vi "NI 5772 (AC) - Digitizer_(FPGA)Averaging (Working)BeforeEdits.vi"() -> ()   [LabVIEW 2020]
doc: "Example Description:\nThis example demonstrates how to enable Time Interleaved Sampling with the NI 5772 adapter module to achieve a sampling rate of 1.6GS/s. This example continuously acquires records of analog input data from the NI 5772 adapter module. It allows you to select an AI channel, trigger type, and record size. This VI must be compiled before it is run. \n\nRunning the VI:\nThis VI must be run from the NI 5772 - Getting Started (Host).vi. Refer to the host VI documentation for steps regarding running and configuring the FPGA VI. \n\nExecution Steps:\nRefer to the Block Diagram of this VI for execution comments."
uses:
  Controls/AI Trigger Type.ctl
  Controls/Aquire State.ctl
  <vilib>/Platform/TimedLoop/XDataNode/timing_clust.ctl
  <vilib>/Platform/TimedLoop/XDataNode/nitl_modes.ctl
  <vilib>/Platform/TimedLoop/XDataNode/wakeup.ctl
  Controls/DigitizerState.ctl
  <vilib>/rvi/Emulation/niFpgaGetClockAttributes.vi
  <vilib>/rvi/Emulation/niFpgaSctlEmulationGetInTimedLoop.vi
  <vilib>/rvi/Emulation/niFpgaEmulationReportErrorSimple.vi
  <vilib>/rvi/eio/common/nirviEmuTemplateMethod_errors.vi
  <vilib>/rvi/Emulation/niFpgaCriticalErrorInLSC.vi
  <vilib>/rvi/Emulation/niFpgaProcessEmulError.vi
  <vilib>/rvi/Emulation/niFpgaEmulationIsFPGAContextNoSignature.vi
  <vilib>/rvi/errors/niFpgaSetErrorForExecOnDevCompSimple.vi
  <vilib>/rvi/eio/common/nirviEmuReportErrorAndStop.vi
  <vilib>/rvi/DataTransferAndStorage/Container/Common/niFpgaContainerGetUniqueNameForEmu.vi
  <vilib>/rvi/FIFO/Fifo_Resource/nirvififoEmulationSetSize.vi
  <vilib>/rvi/FIFO/Fifo_Resource/nirviFifoEmulationQueueMgr.vi
  <instcachedir>/0/nirviFifoEmulationQueueMgr_E5CAEC123FF24DC58D834DCA3CDAA9B5.lvgen/nirviFifoEmulationQueueMgr_E5CAEC123FF24DC58D834DCA3CDAA9B5_000.vi
  <vilib>/Utility/error.llb/Clear Errors.vi
  <vilib>/rvi/FIFO/Fifo_Resource/nirvififoEmulationCreateLock.vi
  <vilib>/rvi/FIFO/Fifo_Resource/nirvififoEmulationObtainLock.vi
  <vilib>/rvi/FIFO/Fifo_Resource/nirvififoEmulationReleaseLock.vi
  <vilib>/rvi/occurrence/nirviWaitOnOccurrenceBase.vi
  <vilib>/rvi/errors/nirviReportUnexpectedCaseInternalError.vi
  <vilib>/rvi/errors/nirviReportUnexpectedCaseInternalError (U32).vi
  <instcachedir>/0/nirviFifoEmulationQueueMgr_E5CAEC123FF24DC58D834DCA3CDAA9B5.lvgen/nirviFifoEmulationQueueMgr_E5CAEC123FF24DC58D834DCA3CDAA9B5_003.vi
  <vilib>/rvi/FIFO/Fifo_Resource/nirvififoEmulationDetermineInputValidOut.vi
  <vilib>/rvi/Memory/Memory_Emulation/nirvimemoryFastEmulation.vi
  <vilib>/rvi/Memory/Memory_Emulation/nirvimemoryEmulation.vi
  <vilib>/rvi/interface/RandomDataEmulation/niFpgaRandomDataHandleErrors.vi
  <instcachedir>/0/nirviFifoEmulationQueueMgr_E5CAEC123FF24DC58D834DCA3CDAA9B5.lvgen/nirviFifoEmulationQueueMgr_E5CAEC123FF24DC58D834DCA3CDAA9B5_004.vi
  <vilib>/eio/EIONode/EIONode.xnode
  <vilib>/Platform/TimedLoop/XDataNode/XDataNode.xnode
  <vilib>/rvi/DataTransferAndStorage/Container/XNode/niFpgaContainer.xnode
  <vilib>/rvi/FIFO/Fifo_Resource/nirvififoEmulationRead.vi
  <vilib>/rvi/FIFO/Fifo_Resource/nirvififoEmulationWrite.vi
  <vilib>/rvi/interface/RandomDataEmulation/nirviRandomDataFpgaReadWriteTemplate.vi
  <vilib>/Platform/TimedLoop/XDataNode/XDNodeRunTimeDep.lvlib
  <instrlib>/_niInstr/Basic Elements/v1/FPGA/niInstr Basic Elements v1 FPGA.lvlib
  <instrlib>/_niInstr/Basic Elements/v1/FPGA/Private/Count Up U64.vi
panel:
  in  "Pulse Width [cycles]":u16=5
  out "Align Wave Counter":u64
  out "Read Size (Host)":u16=512 caption="Samples Per Trigger" min=1 step=1
  out "Trig Count":u64
  in  "TrigIn Simulate":bool
  in  "vi/nGenTrig":bool
  in  "Arm Trigger":bool
  out "F to H FIFO Overflow?":bool caption="FIFO Overflow?"
  out "DataAlignmentFIFO":bool
  out "Aq to Trans FIFO Overflow?":bool caption="FIFO Overflow?"
  in  "Requested Samples Per Pixel":u16=512 caption="Samples Per Trigger" min=1 step=1
  in  "AvgCount_powerOf2":i16=1
  in  "Delay (us)":sgl
  in  "WaveSampleCount":sgl=256.0 format="%#_13g"
  in  "Wave Sampling Rate":sgl=200000000.0 format="%#_6p"
  in  "Trigger Level":i16
  in  "Trigger Type":T1
  out "AvgCount":u16=1
  out "Delay after Trig [cycles]":u16
  out "1/8th Samples Per Trigger":u16=512 caption="Samples Per Trigger" min=1 step=1
  out "WaitForWave\nCompletion [cycles]":u16
  in  "User Command Commit":bool
  in  "User Command":u8
  out "User Command Idle":bool
  out "User Command Status":u8
  in  "User Data 0":u16
  in  "User Data 1":u8
  out "PLL Locked":bool
  out "User Error":bool
  out "Configured?":bool
  # "FIFO Status"
  # "Analog Input"
  # "Resource Configuration"
  # "Clock Configuration"
  # "Trigger Settings"
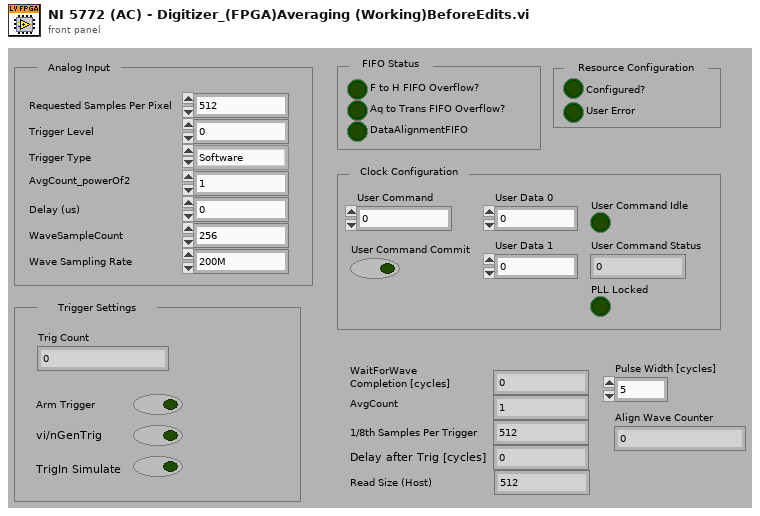
[diagram p1: front panel]
types:
  T1 = typedef "AI Trigger Type.ctl" = enum8{"Software", "Data Edge"}
  T2 = typedef "DigitizerState.ctl" = enum16{"Init", "Build/Clear Accumulator", "GetData", "SetData", "AverageCountCheck", "SendtoHost"}
  T3 = typedef "Aquire State.ctl" = enum8{"Idle", "Wait for Trigger", "AlignWave", "Hold Aquire", "Acquire", "WaitForWaveCompletion", "CheckAvg"}
  T4 = typedef "XDNodeRunTimeDep.lvlib/timing_clust.ctl" = cluster{"Expected End [f-1]":u64, "Actual End [f-1]":u64, "Finished Late? [f-1]":bool, "Expected End [i-1]":u64, "Actual End [i-1]":u64, "Finished Late? [i-1]":bool, "Expected Start [i]":u64, "Actual Start [i]":u64, "Expected Start [f]":u64, "Actual Start [f]":u64, "Source Name":string, "Structure Name":string, "Period":i64, "Deadline":i64, "Offset":i64, "Start":i64, "Priority":i32, "Timeout":i32, "Mode":T5, "Wakeup Reason":T6, "Error":errorcluster, "Source Type":string, "Secondary Source Type":string, "Global End Time":u64, "Global Start Time":u64, "Frame Duration":u64, "Iteration Duration":u64, "Assigned CPU":i32, "I/O Scan Engine Mode":u32}
  T5 = typedef "XDNodeRunTimeDep.lvlib/nitl_modes.ctl" = enum32{"No Change", "Process missed periods, maintain original phase", "Discard missed periods, maintain original phase", "Process missed periods, ignore original phase", "Discard missed periods, ignore original phase"}
  T6 = typedef "XDNodeRunTimeDep.lvlib/wakeup.ctl" = enum32{"Normal", "Aborted", "Asynchronous wakeup", "Timing source error", "Timed loop error", "Timeout"}
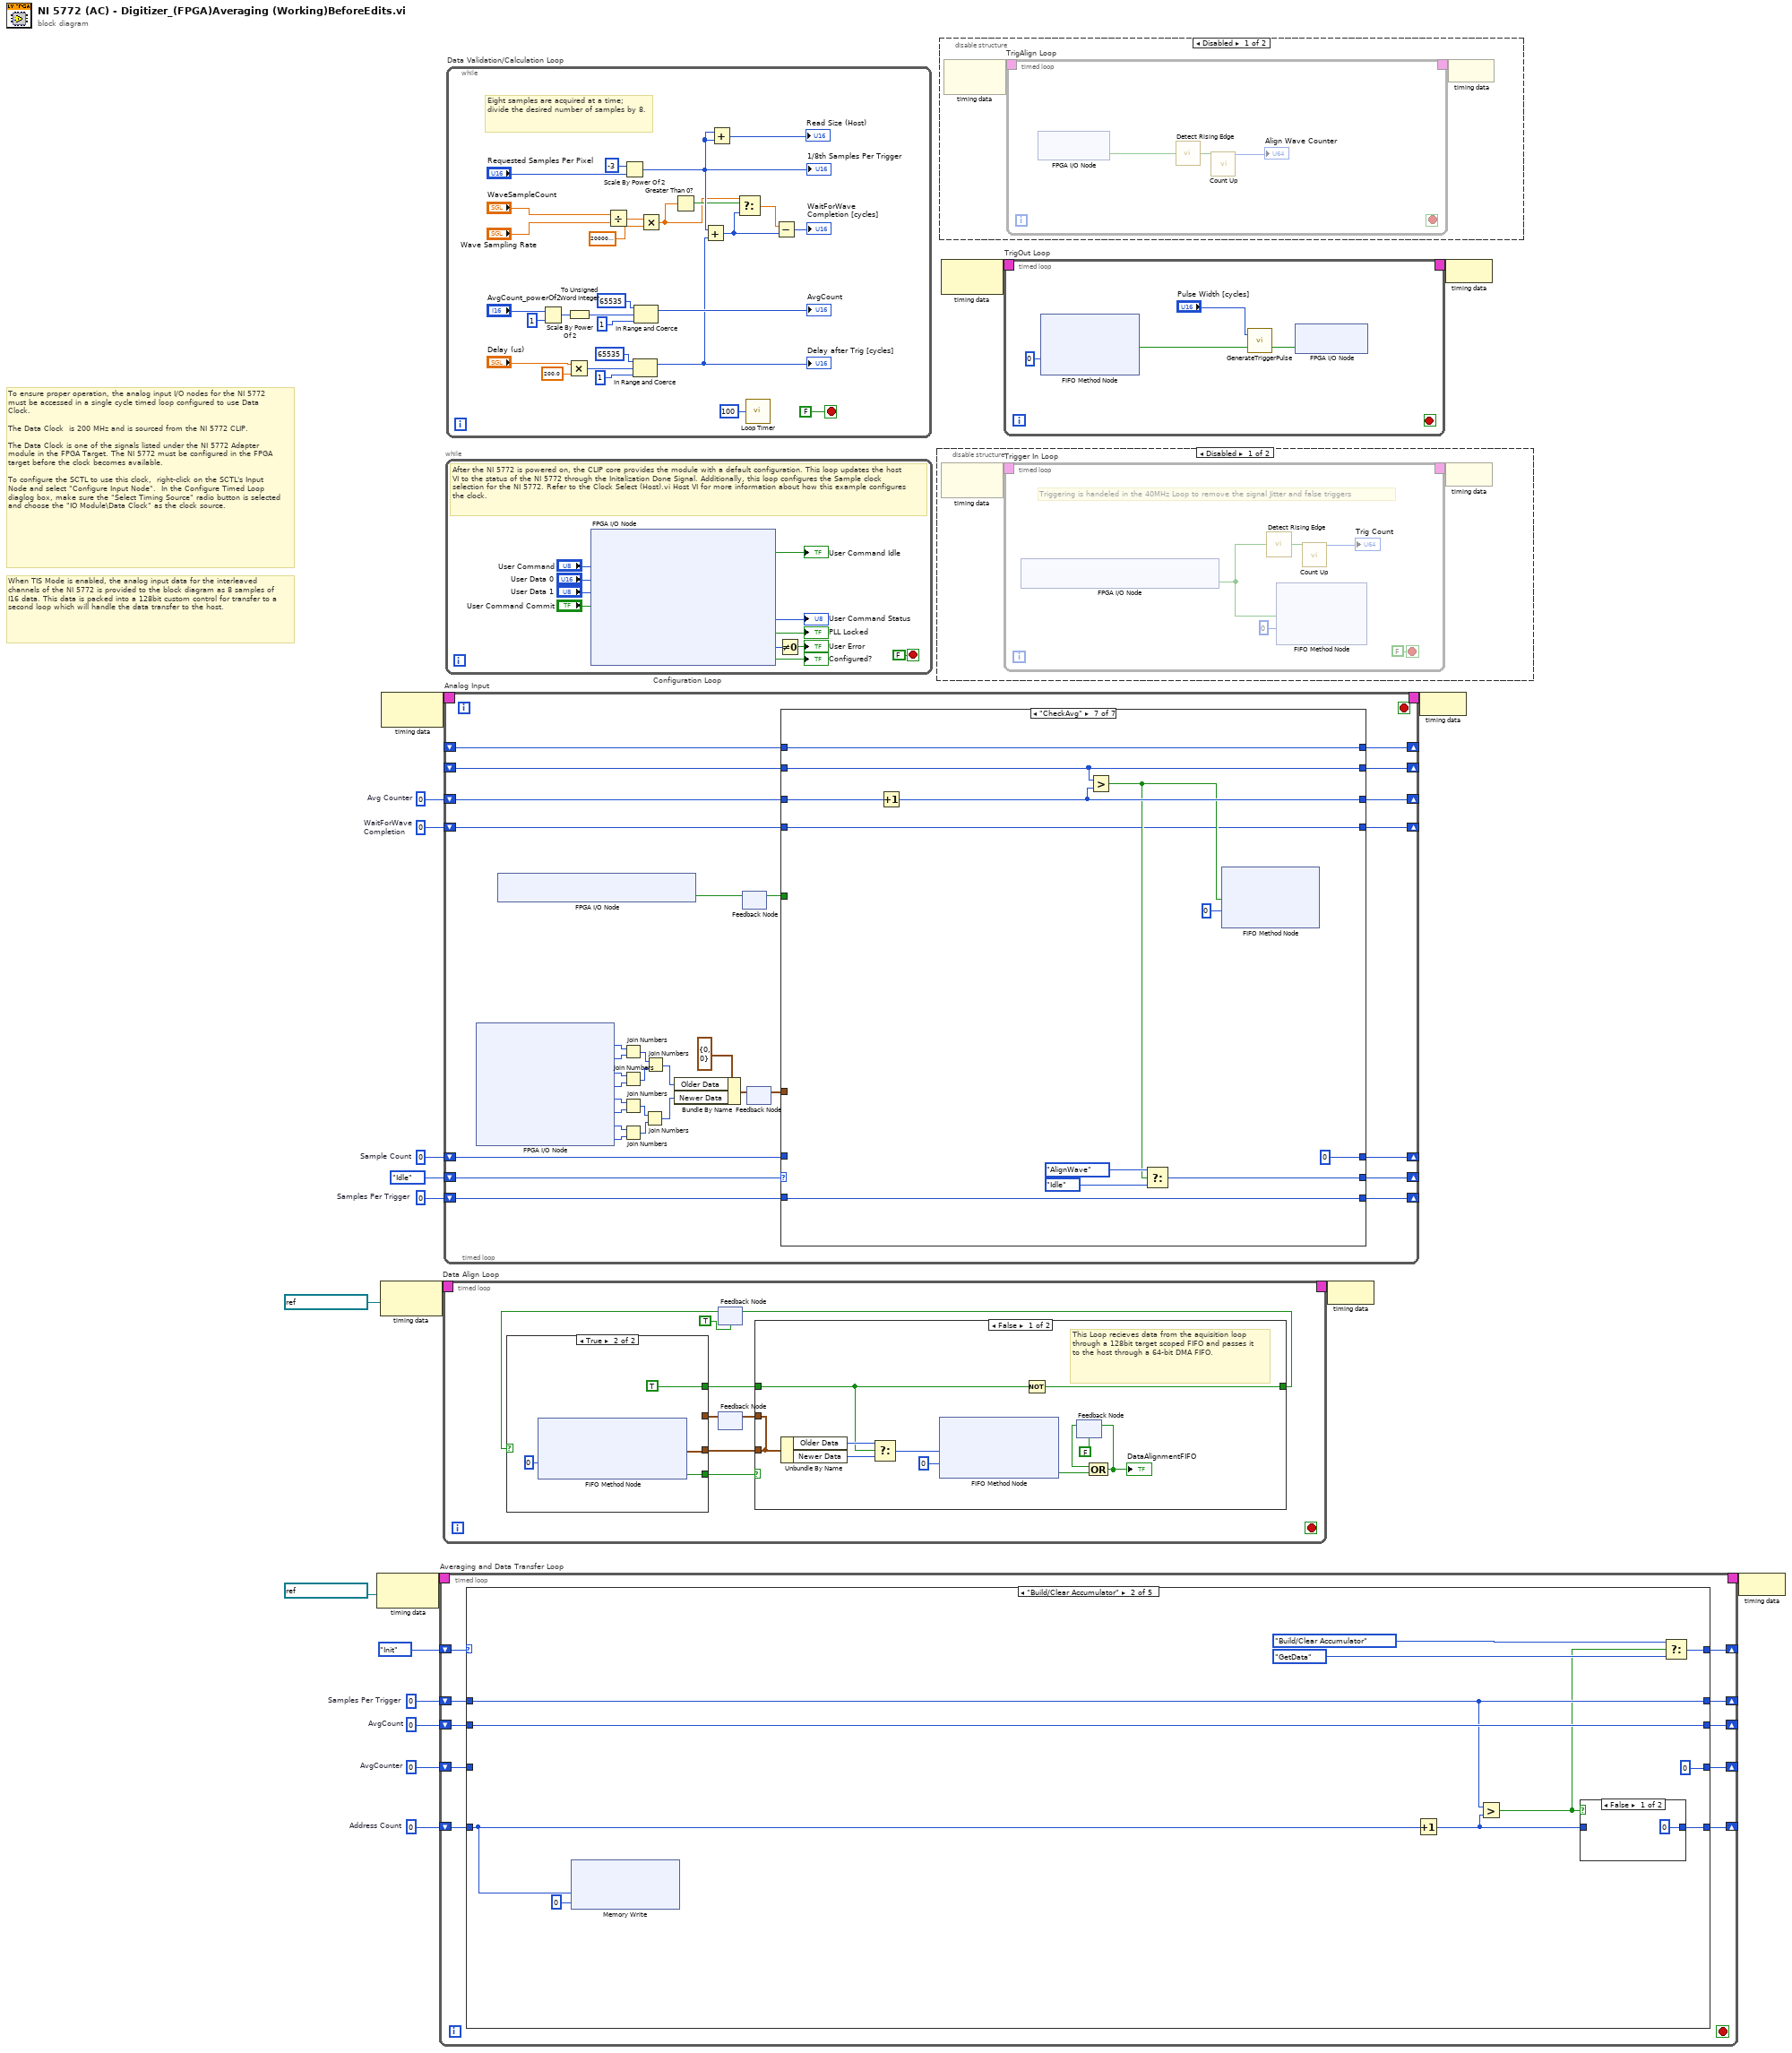
[diagram p0: block diagram]
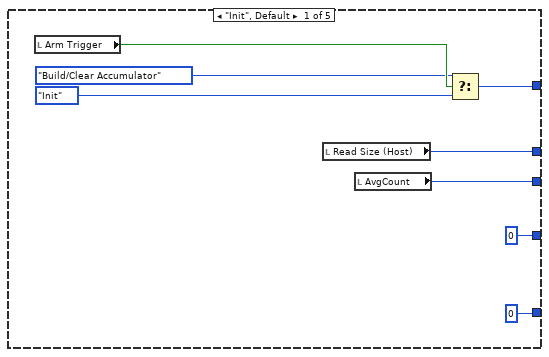
[diagram p4: hidden frame]
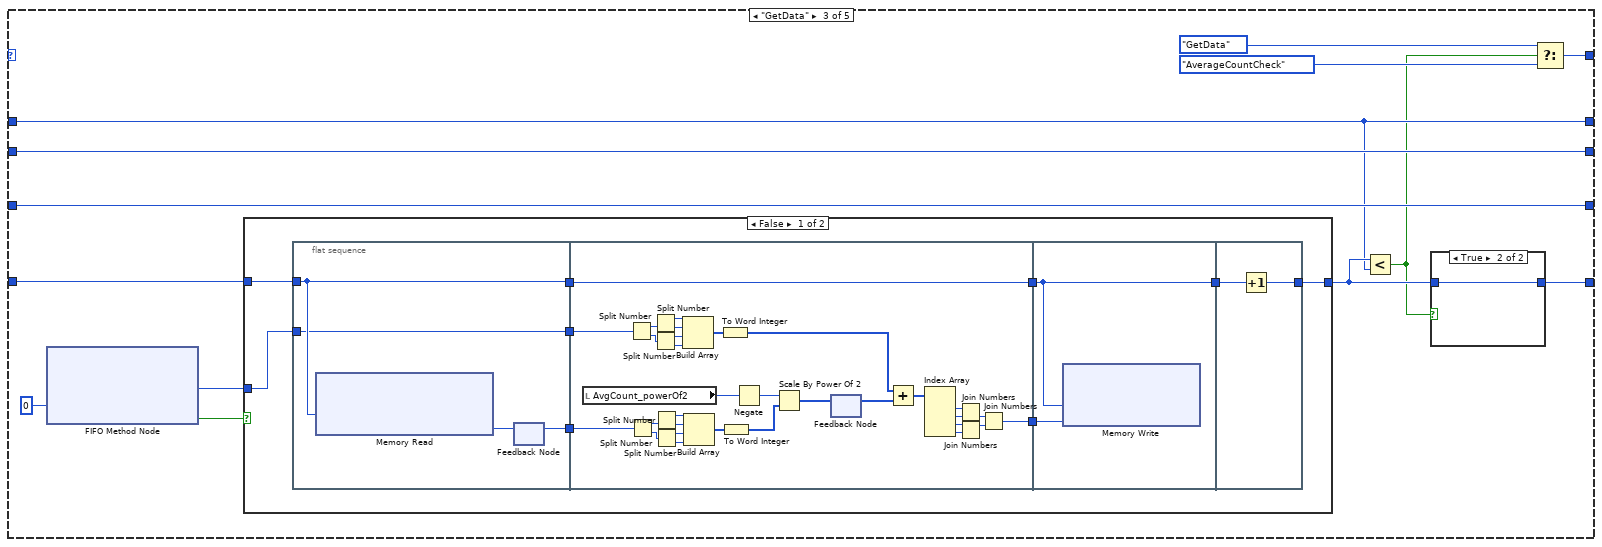
[diagram p6: hidden frame]
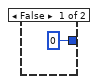
[diagram p7: hidden frame]
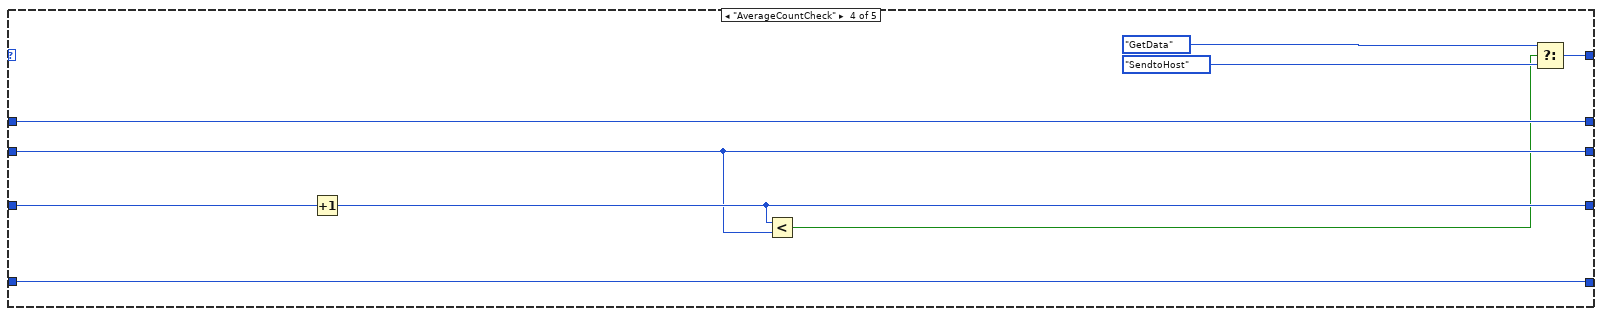
[diagram p9: hidden frame]
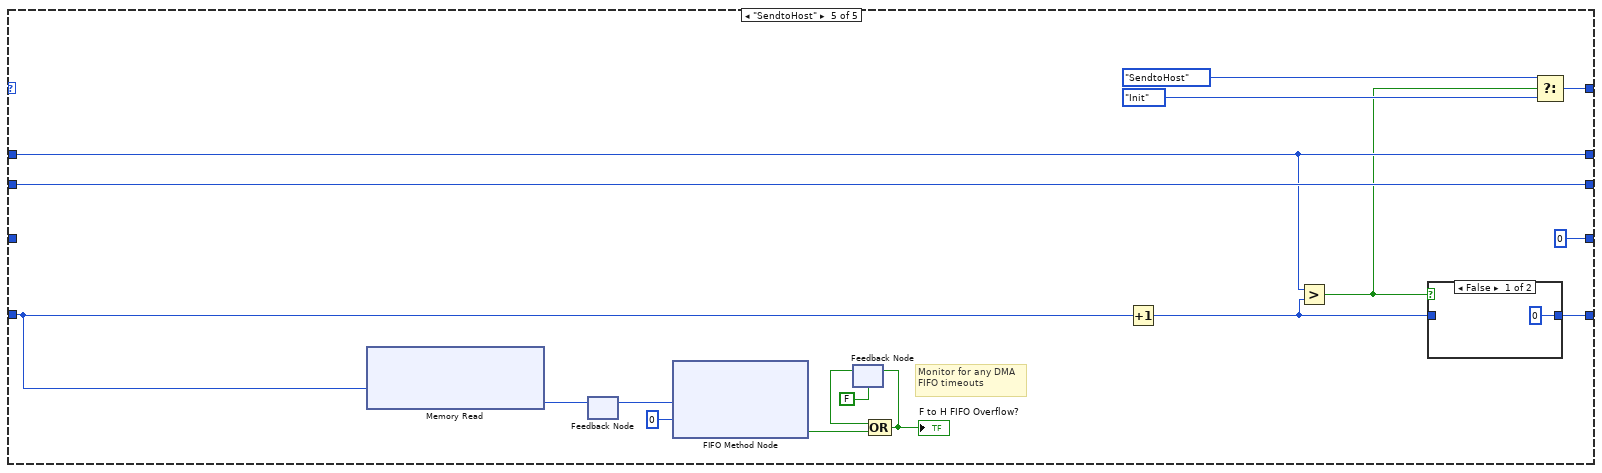
[diagram p10: hidden frame]
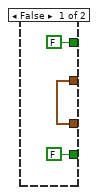
[diagram p12: hidden frame]
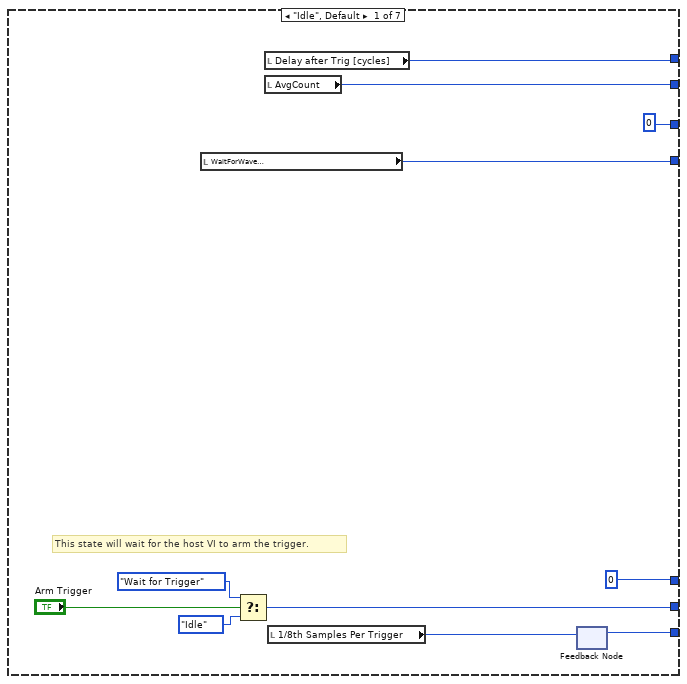
[diagram p14: hidden frame]
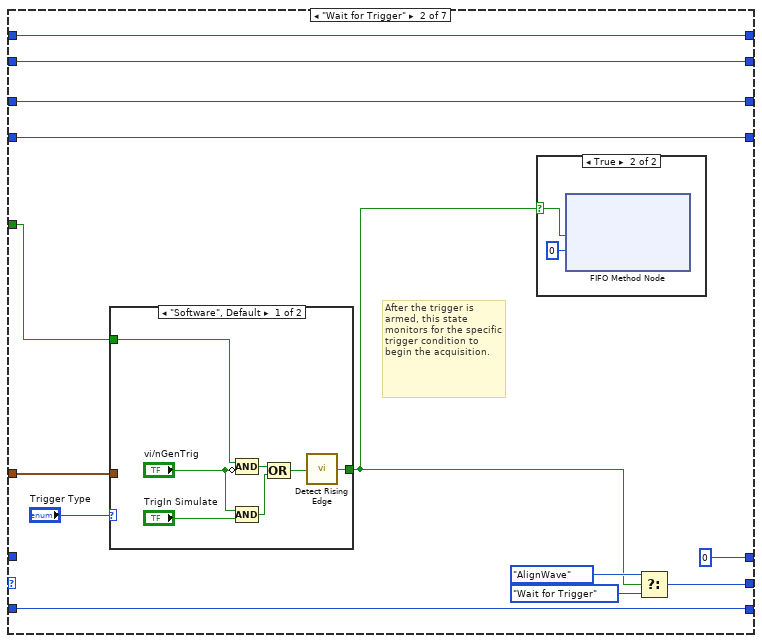
[diagram p15: hidden frame]
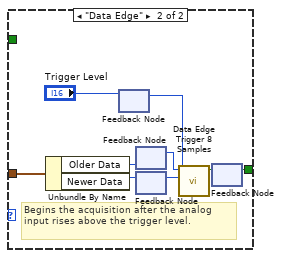
[diagram p17: hidden frame]
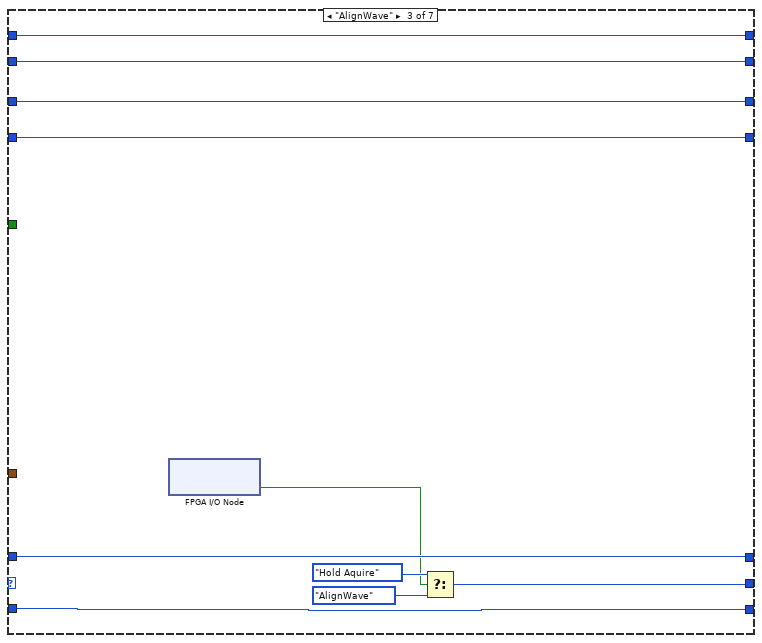
[diagram p18: hidden frame]
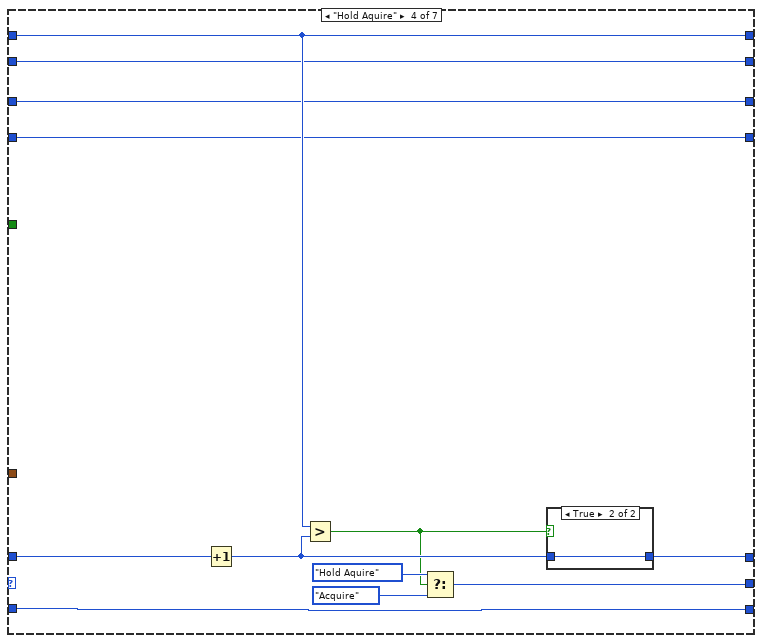
[diagram p19: hidden frame]
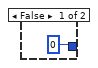
[diagram p20: hidden frame]
diagram:
  w8 = u16 0  # AvgCounter
  w7 = u32 0  # Address Count
  w6 = u16 0  # AvgCount
  w5 = u16 0  # Samples Per Trigger
  w14 = u16 0  # WaitForWave Completion
  w15 = u16 0  # Avg Counter
  w16 = u16 0  # Samples Per Trigger
  w17 = u16 0  # Sample Count
  # "When TIS Mode is enabled, the analog input data for the interleaved channels of the NI 5772 is provided to the block diagram as 8 samples of I16 data. This data is packed into a 128bit custom control for transfer to a second loop which will handle the data transfer to the host."
  # "To ensure proper operation, the analog input I/O nodes for the NI 5772 must be accessed in a single cycle timed loop configured to use Data Clock. \n\nThe Data Clock  is 200 MHz and is sourced from the NI 5772 CLIP.\n\nThe Data Clock is one of the signals listed under the NI 5772 Adapter module in the FPGA Target. The NI 5772 must be configured in the FPGA target before the clock becomes available. \n\nTo configure the SCTL to use this clock,  right-click on the SCTL's Input Node and select \"Configure Input Node\".  In the Configure Timed Loop diaglog box, make sure the \"Select Timing Source\" radio button is selected and choose the \"IO Module\\Data Clock\" as the clock source."
  n1 = node-c288(refnum<k21> "100 MHz Clock" ("Source Name")) -> (w10:T4)
  n2 = node-c288(refnum<k21> "100 MHz Clock" ("Source Name")) -> (w13:T4)
  n3 = node-c288() -> (w20:T4)  [unwired: 1 in]
  n4 = timed-loop "Averaging and Data Transfer Loop" {
    timing: w10 -> [_]
    timing-out: [_] -> w9
    shift-right: [w29] -> _
    shift-left: DigitizerState."Init" -> [w30]
    shift-right: [w28] -> _
    shift-left: w5 -> [w26]
    shift-right: [w27] -> _
    shift-left: w6 -> [w25]
    shift-right: [w23] -> _
    shift-left: w7 -> [w24]
    shift-right: [w21] -> _
    shift-left: w8 -> [w22]
    stop <- _ stop-if-true
    n5 = case shown="\"Build/Clear Accumulator\"" w30 {
      tunnel: [w34 w46 w62 w122 w138] -> w29
      tunnel: [w32 w44 w54 w120 w136] -> w28
      tunnel: [w35 w49 w61 w117 w141] -> w27
      tunnel: w26 -> [_ w44 w54 w120 w136]
      tunnel: w25 -> [_ w49 w61 w117 w141]
      tunnel: w24 -> [_ w40 w57 w121 w126]
      tunnel: [u32 0 w45 w56 w121 w137] -> w23
      tunnel: [u16 0 u16 0 ("AvgCounter") w59 w118 u16 0 ("AvgCounter")] -> w21
      tunnel: w22 -> [_ _ w59 w119 _]
      frame "Init", Default {
        n6 = local read "Arm Trigger"() -> (w38:bool)
        n7 = local read "Read Size (Host)"() -> (w32:u16)
        n8 = local read "AvgCount"() -> (w35:u16)
        n9 = Select(t=DigitizerState."Build/Clear Accumulator", s=w38, f=DigitizerState."Init") -> (s? t:f=w34:T2)
      }
      frame "Build/Clear Accumulator" {
        n10 = xnode ("Memory Write")("Address"=w40, "Data"=u64 0) -> ()  [unwired: 1 in, 1 out]
        n11 = Increment(x=w40) -> (x+1=w43:u32)
        n12 = Greater?(x=w44, y=w43) -> (0:w42:bool)
        n13 = case shown="False" w42 {
          tunnel: w43 -> [_ w51]
          tunnel: [u32 0 w51] -> w45
          frame False {
          }
          frame True {
          }
        }
        n14 = Select(t=DigitizerState."Build/Clear Accumulator", s=w42, f=DigitizerState."GetData") -> (s? t:f=w46:T2)
      }
      frame "GetData" {
        n15 = xnode ("FIFO Method Node")("Timeout"=0) -> ("Element"=w58:u64, "Timed Out?"=w53:bool)  [unwired: 1 in, 1 out]
        n16 = case shown="False" w53 {
          tunnel: w58 -> [w72 _]
          tunnel: w57 -> [w74 w115]
          tunnel: [w71 w115] -> w55
          frame False {
            n17 = flat-sequence {
              tunnel: [w78] -> w75
              tunnel: w74 -> [w77]
              tunnel: w72 -> [w76]
              tunnel: [w77] -> w70
              tunnel: [w76] -> w68
              tunnel: w75 -> [w81]
              tunnel: [w100] -> w73
              tunnel: w70 -> [w99]
              tunnel: [w99] -> w69
              tunnel: w68 -> [w90]
              tunnel: w73 -> [w112]
              tunnel: w69 -> [w111]
              tunnel: [w111] -> w67
              tunnel: [w113] -> w71
              tunnel: w67 -> [w114]
              frame #0 {
                n18 = xnode ("Memory Read")("Address"=w77) -> ("Data"=w79:u64)  [unwired: 1 in, 1 out]
                n19 = feedback #1() -> (w78:u64)  [unwired: 1 in]
                n20 = feedback-in #1(w79) -> ()
              }
              frame #1 {
                n21 = local read "AvgCount_powerOf2"() -> (w109:i16)
                n22 = Split Number(x=w90) -> (hi(x)=w97:u32, lo(x)=w96:u32)
                n23 = Split Number(x=w81) -> (hi(x)=w82:u32, lo(x)=w83:u32)
                n24 = Split Number(x=w97) -> (hi(x)=w95:u16, lo(x)=w94:u16)
                n25 = Split Number(x=w96) -> (hi(x)=w93:u16, lo(x)=w92:u16)
                n26 = Split Number(x=w82) -> (hi(x)=w84:u16, lo(x)=w85:u16)
                n27 = Split Number(x=w83) -> (hi(x)=w86:u16, lo(x)=w87:u16)
                n28 = Build Array(w95, w94, w93, w92) -> (w91:u16[])
                n29 = Build Array(w84, w85, w86, w87) -> (w88:u16[])
                n30 = To Word Integer(number=w91) -> (16bit integer=w89:i16[])
                n31 = To Word Integer(number=w88) -> (16bit integer=w80:i16[])
                n32 = Negate(x=w109) -> (-x=w110:i16)
                n33 = Scale By Power Of 2(n=w110, x=w80) -> (x*2^n=w108:i16[])
                n34 = feedback-in #2(w108) -> ()
                n35 = feedback #2() -> (w98:i16[])  [unwired: 1 in]
                n36 = Add(x=w89, y=w98) -> (x+y=w101:i16[])
                n37 = Index Array(array=w101) -> (element #1=w104:i16, element #2=w105:i16, element #3=w106:i16, element #4=w107:i16)  [unwired: 4 in]
                n38 = Join Numbers(hi=w104, lo=w105) -> ((hi.lo)=w102:u32)
                n39 = Join Numbers(hi=w106, lo=w107) -> ((hi.lo)=w103:u32)
                n40 = Join Numbers(hi=w102, lo=w103) -> ((hi.lo)=w100:u64)
              }
              frame #2 {
                n41 = xnode ("Memory Write")("Address"=w111, "Data"=w112) -> ()  [unwired: 1 in, 1 out]
              }
              frame #3 {
                n42 = Increment(x=w114) -> (x+1=w113:u32)
              }
            }
          }
          frame True {
          }
        }
        n43 = Less?(x=w55, y=w54) -> (x < y?=w52:bool)
        n44 = case shown="True" w52 {
          tunnel: w55 -> [_ w66]
          tunnel: [u32 0 w66] -> w56
          frame False {
          }
          frame True {
          }
        }
        n45 = Select(t=DigitizerState."GetData", s=w52, f=DigitizerState."AverageCountCheck") -> (s? t:f=w62:T2)
      }
      frame "AverageCountCheck" {
        n46 = Increment(x=w119) -> (x+1=w118:u16)
        n47 = Less?(x=w118, y=w117) -> (x < y?=w116:bool)
        n48 = Select(t=DigitizerState."GetData", s=w116, f=DigitizerState."SendtoHost") -> (s? t:f=w122:T2)
      }
      frame "SendtoHost" {
        # "Monitor for any DMA FIFO timeouts"
        n49 = xnode ("Memory Read")("Address"=w126) -> ("Data"=w127:u64)  [unwired: 1 in, 1 out]
        n50 = feedback #3() -> (w125:u64)  [unwired: 1 in]
        n51 = feedback-in #3(w127) -> ()
        n52 = xnode ("FIFO Method Node")("Element"=w125, "Timeout"=0) -> ("Timed Out?"=w132:bool)  [unwired: 1 in, 1 out]
        n53 = feedback #4(FALSE) -> (w131:bool)
        n54 = Compound Arithmetic op=OR(w131, w132) -> (w133:bool)
        "F to H FIFO Overflow?" <- w133
        n55 = feedback-in #4(w133) -> ()
        n56 = Increment(x=w126) -> (x+1=w135:u32)
        n57 = Greater?(x=w136, y=w135) -> (0:w134:bool)
        n58 = case shown="False" w134 {
          tunnel: w135 -> [_ w143]
          tunnel: [u32 0 w143] -> w137
          frame False {
          }
          frame True {
          }
        }
        n59 = Select(t=DigitizerState."SendtoHost", s=w134, f=DigitizerState."Init") -> (s? t:f=w138:T2)
      }
    }
  }
  n60 = timed-loop "Data Align Loop" {
    timing: w13 -> [_]
    timing-out: [_] -> w12
    stop <- _ stop-if-true
    n61 = feedback #5(TRUE ("Timed Out?")) -> (w148:bool)
    n62 = feedback #6() -> (w149:cluster{"Older Data":u64, "Newer Data":u64})  [unwired: 1 in]
    n63 = case shown="True" w148 {
      tunnel: [w154 w157] -> w151
      tunnel: [FALSE ("Timed Out?") w158] -> w153
      tunnel: [FALSE ("Timed Out?") TRUE ("Timed Out?")] -> w152
      tunnel: w149 -> [w154 _]
      frame False {
      }
      frame True {
        n64 = xnode ("FIFO Method Node")("Timeout"=0) -> ("Element"=w157:cluster{"Older Data":u64, "Newer Data":u64}, "Timed Out?"=w158:bool)  [unwired: 1 in, 1 out]
      }
    }
    n65 = case shown="False" w153 {
      tunnel: [w169 w173] -> w147
      tunnel: w152 -> [w170 w173]
      tunnel: w151 -> [w168 w172]
      tunnel: [w168 w172] -> w150
      frame False {
        # "This Loop recieves data from the aquisition loop through a 128bit target scoped FIFO and passes it to the host through a 64-bit DMA FIFO."
        n66 = Unbundle By Name(w168) -> ("Older Data"=w171:u64, "Newer Data"=w167:u64)
        n67 = Select(t=w171, s=w170, f=w167) -> (s? t:f=w161:u64)
        n68 = xnode ("FIFO Method Node")("Element"=w161, "Timeout"=0) -> ("Timed Out?"=w163:bool)  [unwired: 1 in, 1 out]
        n69 = Not(x=w170) -> (.not. x?=w169:bool)
        n70 = feedback #7(FALSE) -> (w164:bool)
        n71 = Compound Arithmetic op=OR(w164, w163) -> (w162:bool)
        "DataAlignmentFIFO" <- w162
        n72 = feedback-in #7(w162) -> ()
      }
      frame True {
      }
    }
    n73 = feedback-in #5(w147) -> ()
    n74 = feedback-in #6(w150) -> ()
  }
  n75 = timed-loop "Analog Input" {
    timing: w20 -> [_]
    timing-out: [_] -> w19
    shift-right: [w207] -> _
    shift-left: Aquire_State."Idle" ("Acquire State") -> [w197]
    shift-right: [w208] -> _
    shift-left: w17 -> [w198]
    shift-right: [w206] -> _
    shift-left: w16 -> [w196]
    shift-right: [w184] -> _
    shift-left: _ -> [w183]
    shift-right: [w182] -> _
    shift-left: _ -> [w181]
    shift-right: [w179] -> _
    shift-left: w15 -> [w180]
    shift-right: [w178] -> _
    shift-left: w14 -> [w177]
    stop <- _ stop-if-true
    n76 = xnode "FPGA I/O Node"() -> ("IO Module\\AI 1 Data N-3"=w189:i16, "IO Module\\AI 0 Data N-3"=w188:i16, "IO Module\\AI 1 Data N-2"=w187:i16, "IO Module\\AI 0 Data N-2"=w186:i16, "IO Module\\AI 1 Data N-1"=w190:i16, "IO Module\\AI 0 Data N-1"=w191:i16, "IO Module\\AI 1 Data N"=w192:i16, "IO Module\\AI 0 Data N"=w193:i16)  [unwired: 8 in, 8 out]
    n77 = xnode "FPGA I/O Node"() -> ("IO Module\\Asynchronous Trigger Input"=w185:bool)  [unwired: 1 in, 1 out]
    n78 = Join Numbers(hi=w189, lo=w188) -> ((hi.lo)=w201:u32)
    n79 = Join Numbers(hi=w187, lo=w186) -> ((hi.lo)=w203:u32)
    n80 = Join Numbers(hi=w190, lo=w191) -> ((hi.lo)=w202:u32)
    n81 = Join Numbers(hi=w192, lo=w193) -> ((hi.lo)=w204:u32)
    n82 = Join Numbers(hi=w202, lo=w204) -> ((hi.lo)=w194:u64)
    n83 = Join Numbers(hi=w201, lo=w203) -> ((hi.lo)=w195:u64)
    n84 = Bundle By Name(cluster=cluster{"Older Data":u64, "Newer Data":u64} {"Older Data"=0, "Newer Data"=0} ("Element"), "Older Data"=w195, "Newer Data"=w194) -> (w199:cluster{"Older Data":u64, "Newer Data":u64})
    n85 = feedback-in #8(w185) -> ()
    n86 = feedback #8() -> (w176:bool)  [unwired: 1 in]
    n87 = feedback #9() -> (w205:cluster{"Older Data":u64, "Newer Data":u64})  [unwired: 1 in]
    n88 = feedback-in #9(w199) -> ()
    n89 = case shown="\"CheckAvg\"" w197 {
      tunnel: [u16 0 u16 0 w256 w268 w278 w296 u16 0] -> w208
      tunnel: w198 -> [_ _ w256 w267 w289 w298 _]
      tunnel: [w216 w228 w259 w271 w288 w301 w312] -> w207
      tunnel: [w214 w232 w257 w269 w285 w299 w310] -> w206
      tunnel: w196 -> [_ w232 w257 w269 w285 w299 w310]
      tunnel: w205 -> [_ w231 _ _ w284 _ _]
      tunnel: w176 -> [_ w226 _ _ _ _ _]
      tunnel: [w213 w225 w255 w266 w282 w297 w309] -> w184
      tunnel: w183 -> [_ w225 w255 w266 w282 w297 w309]
      tunnel: [w212 w224 w254 w264 w281 w294 w307] -> w182
      tunnel: w181 -> [_ w224 w254 w264 w281 w294 w307]
      tunnel: [u16 0 ("Avg Count") w223 w253 w263 w280 w293 w306] -> w179
      tunnel: w180 -> [_ w223 w253 w263 w280 w293 w308]
      tunnel: [w209 w221 w252 w261 w276 w292 w303] -> w178
      tunnel: w177 -> [_ w221 w252 w261 w276 w292 w303]
      frame "Idle", Default {
        # "This state will wait for the host VI to arm the trigger."
        n90 = local read "WaitForWave\nCompletion [cycles]"() -> (w209:u16)
        n91 = Select(t=Aquire_State."Wait for Trigger" ("Acquire State"), s="Arm Trigger", f=Aquire_State."Idle" ("Acquire State")) -> (s? t:f=w216:T3)
        n92 = local read "Delay after Trig [cycles]"() -> (w213:u16)
        n93 = local read "AvgCount"() -> (w212:u16)
        n94 = local read "1/8th Samples Per Trigger"() -> (w210:u16)
        n95 = feedback-in #10(w210) -> ()
        n96 = feedback #10() -> (w214:u16)  [unwired: 1 in]
      }
      frame "Wait for Trigger" {
        # "After the trigger is armed, this state monitors for the specific trigger condition to begin the acquisition."
        n97 = case shown="\"Software\", Default" "Trigger Type" {
          tunnel: w231 -> [_ w250]
          tunnel: [w241 w242] -> w222
          tunnel: w226 -> [w236 _]
          frame "Software", Default {
            n98 = Compound Arithmetic op=AND(w236, invert "vi/nGenTrig") -> (w240:bool)
            n99 = Compound Arithmetic op=AND("vi/nGenTrig", "TrigIn Simulate") -> (w238:bool)
            n100 = Compound Arithmetic op=OR(w240, w238) -> (w235:bool)
            n101 = call <instrlib>:"Detect Rising Edge.vi"("signal"=w235) -> ("edge detected"=w241:bool)  [unwired: 14 in]
          }
          frame "Data Edge" {
            # "Begins the acquisition after the analog input rises above the trigger level."
            n102 = Unbundle By Name(w250) -> ("Older Data"=w248:u64, "Newer Data"=w246:u64)
            n103 = feedback-in #11("Trigger Level") -> ()
            n104 = feedback #11() -> (w244:i16)  [unwired: 1 in]
            n105 = feedback-in #12(w248) -> ()
            n106 = feedback #12() -> (w243:u64)  [unwired: 1 in]
            n107 = feedback-in #13(w246) -> ()
            n108 = feedback #13() -> (w245:u64)  [unwired: 1 in]
            n109 = call "Data Edge Trigger 8 Samples.vi"("Trigger Level"=w244, "Newer Data In"=w245, "Older Data In"=w243) -> ("Trigger"=w249:bool)  [unwired: 8 in]
            n110 = feedback-in #14(w249) -> ()
            n111 = feedback #14() -> (w242:bool)  [unwired: 1 in]
          }
        }
        n112 = case shown="True" w222 {
          selector: w222 -> [_ w234]
          frame False {
          }
          frame True {
            n113 = xnode ("FIFO Method Node")("Element"=w234, "Timeout"=0) -> ()  [unwired: 1 in, 2 out]
          }
        }
        n114 = Select(t=Aquire_State."AlignWave" ("Acquire State"), s=w222, f=Aquire_State."Wait for Trigger") -> (s? t:f=w228:T3)
      }
      frame "AlignWave" {
        n115 = xnode "FPGA I/O Node"() -> ("PXI_Trig0"=w251:bool)  [unwired: 1 in, 1 out]
        n116 = Select(t=Aquire_State."Hold Aquire" ("Acquire State"), s=w251, f=Aquire_State."AlignWave" ("Acquire State")) -> (s? t:f=w259:T3)
      }
      frame "Hold Aquire" {
        n117 = Increment(x=w267) -> (x+1=w265:u16)
        n118 = Greater?(x=w266, y=w265) -> (0:w262:bool)
        n119 = Select(t=Aquire_State."Hold Aquire" ("Acquire State"), s=w262, f=Aquire_State."Acquire" ("Acquire State")) -> (s? t:f=w271:T3)
        n120 = case shown="True" w262 {
          tunnel: [u16 0 w274] -> w268
          tunnel: w265 -> [_ w274]
          frame False {
          }
          frame True {
          }
        }
      }
      frame "Acquire" {
        # "Monitor for any  FIFO timeouts"
        # "While in this state, data is pushed into a DMA FIFO until the desired number of samples per record have been acquired."
        n121 = xnode ("FIFO Method Node")("Element"=w284, "Timeout"=0) -> ("Timed Out?"=→"Aq to Trans FIFO Overflow?":bool)  [unwired: 1 in, 1 out]
        n122 = Increment(x=w289) -> (x+1=w279:u16)
        n123 = Less?(x=w279, y=w285) -> (x < y?=w277:bool)
        n124 = Select(t=Aquire_State."Acquire" ("Acquire State"), s=w277, f=Aquire_State."WaitForWaveCompletion" ("Acquire State")) -> (s? t:f=w288:T3)
        n125 = case shown="False" w277 {
          tunnel: w279 -> [_ w291]
          tunnel: [u16 0 w291] -> w278
          frame False {
          }
          frame True {
          }
        }
      }
      frame "WaitForWaveCompletion" {
        n126 = Increment(x=w298) -> (x+1=w296:u16)
        n127 = Greater?(x=w292, y=w296) -> (0:w295:bool)
        n128 = Select(t=Aquire_State."WaitForWaveCompletion" ("Acquire State"), s=w295, f=Aquire_State."CheckAvg" ("Acquire State")) -> (s? t:f=w301:T3)
      }
      frame "CheckAvg" {
        n129 = Increment(x=w308) -> (x+1=w306:u16)
        n130 = Greater?(x=w307, y=w306) -> (0:w304:bool)
        n131 = Select(t=Aquire_State."AlignWave" ("Acquire State"), s=w304, f=Aquire_State."Idle") -> (s? t:f=w312:T3)
        n132 = xnode ("FIFO Method Node")("Element"=w304, "Timeout"=0) -> ()  [unwired: 1 in, 2 out]
      }
    }
  }
  n133 = while "Configuration Loop" {
    stop <- FALSE stop-if-true
    # "After the NI 5772 is powered on, the CLIP core provides the module with a default configuration. This loop updates the host VI to the status of the NI 5772 through the Initalization Done Signal. Additionally, this loop configures the Sample clock selection for the NI 5772. Refer to the Clock Select (Host).vi Host VI for more information about how this example configures the clock."
    n134 = xnode "FPGA I/O Node"("IO Module\\User Command"="User Command", "IO Module\\User Data 0"="User Data 0", "IO Module\\User Data 1"="User Data 1", "IO Module\\User Command Commit"="User Command Commit") -> ("IO Module\\User Command Idle"=→"User Command Idle":bool, "IO Module\\User Command Status"=→"User Command Status":u8, "IO Module\\PLL Locked"=→"PLL Locked":bool, "IO Module\\User Error"=w322:u8, "IO Module\\Initialization Done"=→"Configured?":bool)  [unwired: 9 in, 9 out]
    n135 = Not Equal To 0?(x=w322) -> (x != 0?=→"User Error":bool)
  }
  n136 = while "Data Validation/Calculation Loop" {
    stop <- FALSE stop-if-true
    # "Eight samples are acquired at a time; divide the desired number of samples by 8."
    n137 = Scale By Power Of 2(n="AvgCount_powerOf2", x=1 ("Timeout")) -> (x*2^n=w353:i32)
    n138 = To Unsigned Word Integer(number=w353) -> (unsigned 16bit integer=w350:u16)
    n139 = Multiply(x="Delay (us)", y=sgl 200.0) -> (x*y=w346:u16)
    n140 = Divide(x="WaveSampleCount", y="Wave Sampling Rate") -> (x/y=w338:sgl)
    n141 = Scale By Power Of 2(n=i16 -3, x="Requested Samples Per Pixel") -> (x*2^n=w332:u16)
    "1/8th Samples Per Trigger" <- w332
    n142 = In Range and Coerce(upper limit=u16 65535, x=w346, lower limit=u16 1) -> (coerced(x)=w339:u16)  [unwired: 1 out]
    "Delay after Trig [cycles]" <- w339
    n143 = In Range and Coerce(upper limit=u16 65535, x=w350, lower limit=u16 1) -> (coerced(x)=→"AvgCount":u16)  [unwired: 1 out]
    n144 = Multiply(x=w338, y=sgl 200000000.0) -> (x*y=w329:sgl)
    n145 = Greater Than 0?(x=w329) -> (x > 0?=w330:bool)
    n146 = Add(x=w332, y=w339) -> (x+y=w328:u16)
    n147 = Add(x=w332, y=w332) -> (x+y=→"Read Size (Host)":u16)
    n148 = Select(t=w329, s=w330, f=w328) -> (s? t:f=w331:sgl)
    n149 = call "Loop Timer"("Count(uSec)"=u32 100 ("Count(mSec)")) -> ()  [unwired: 1 out]
    n150 = Subtract(x=w331, y=w328) -> (x-y=→"WaitForWave\nCompletion [cycles]":u16)
  }
  n151 = disable-structure shown="Disabled" {
    frame Disabled {
      n152 = node-c288() -> (w357:T4)  [unwired: 1 in]
      n153 = timed-loop "Trigger In Loop" {
        timing: w357 -> [_]
        timing-out: [_] -> w356
        stop <- FALSE stop-if-true
        # "Triggering is handeled in the 40MHz Loop to remove the signal Jitter and false triggers"
        n154 = xnode "FPGA I/O Node"() -> ("IO Module\\Asynchronous Trigger Input"=w362:bool)  [unwired: 1 in, 1 out]
        n155 = call <instrlib>:"Detect Rising Edge.vi"("signal"=w362) -> ("edge detected"=w359:bool)  [unwired: 14 in]
        n156 = xnode ("FIFO Method Node")("Element"=w362, "Timeout"=0) -> ()  [unwired: 1 in, 2 out]
        n157 = call-poly <instrlib>:"Count Up.vi"("increment"=w359) -> ("count out"=→"Trig Count":u64)  [unwired: 14 in]
      }
      n158 = node-c288(w356) -> ()
    }
    frame Enabled {
    }
  }
  n159 = disable-structure shown="Disabled" {
    frame Disabled {
      n160 = node-c288() -> (w368:T4)  [unwired: 1 in]
      n161 = timed-loop "TrigAlign Loop" {
        timing: w368 -> [_]
        timing-out: [_] -> w367
        stop <- _ stop-if-true
        n162 = xnode "FPGA I/O Node"() -> ("PXI_Trig0"=w369:bool)  [unwired: 1 in, 1 out]
        n163 = call <instrlib>:"Detect Rising Edge.vi"("signal"=w369) -> ("edge detected"=w370:bool)  [unwired: 14 in]
        n164 = call-poly <instrlib>:"Count Up.vi"("increment"=w370) -> ("count out"=→"Align Wave Counter":u64)  [unwired: 14 in]
      }
      n165 = node-c288(w367) -> ()
    }
    frame Enabled {
    }
  }
  n166 = node-c288() -> (w2:T4)  [unwired: 1 in]
  n167 = timed-loop "TrigOut Loop" {
    timing: w2 -> [_]
    timing-out: [_] -> w1
    stop <- _ stop-if-true
    n168 = xnode ("FIFO Method Node")("Timeout"=0) -> ("Element"=w377:bool)  [unwired: 1 in, 2 out]
    n169 = call "GenerateTriggerPulse.vi"("Trigger"=w377, "Pulse Width [cycles]"="Pulse Width [cycles]") -> ("Out"=w378:bool)  [unwired: 1 out]
    n170 = xnode "FPGA I/O Node"("PXI_Trig1"=w378) -> ()  [unwired: 1 in, 1 out]
  }
  n171 = node-c288(w12) -> ()
  n172 = node-c288(w19) -> ()
  n173 = node-c288(w1) -> ()
  n174 = node-c288(w9) -> ()
